vi "SubVI_SingleWrite.vi"() -> ()   [LabVIEW 2022 SP3, in "ADS_Library.lvlib"]
uses:
  ADS_Library.lvlib
  <userlib>/Beckhoff-LabVIEW-Interface/_DependsOn/Base/Write/Write Sync.vi
panel:
  in  "Ads Write Data":variant
  out "Write Status":bool
  out "SymbolName":string
  out "error out":errorcluster
  in  "error in":errorcluster
  in  "String":string
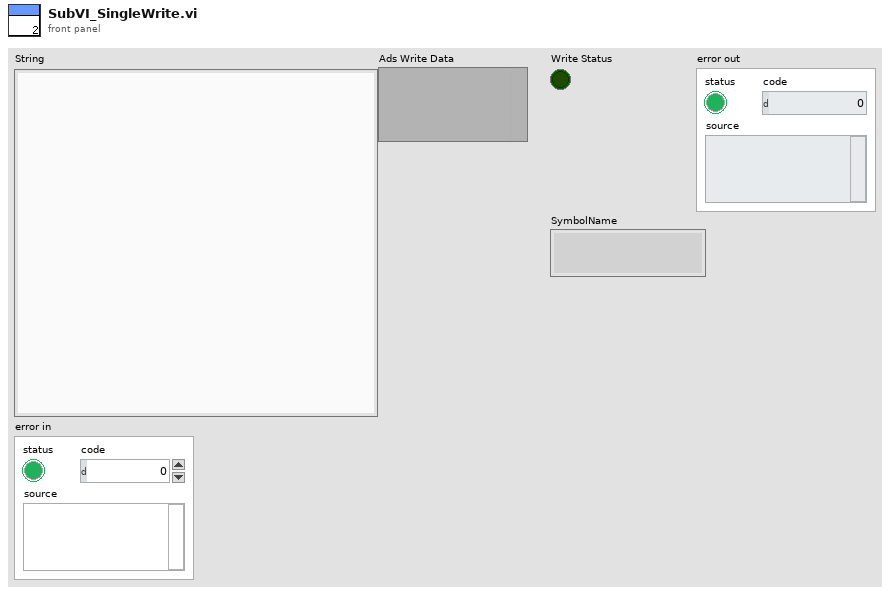
[diagram p1: front panel]
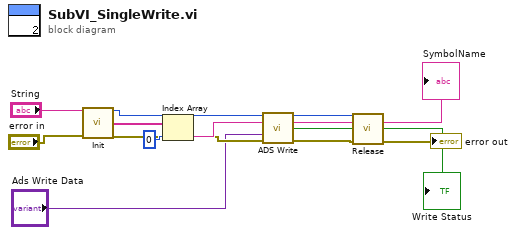
[diagram p0: block diagram]
diagram:
  n1 = call <userlib>:"Init.vi"("XMLDescription"="String", "error in (no error)"="error in") -> ("Handle"=w8:u32, "ReadGrpSymbols"=w12:string[], "error out"=w6:errorcluster)  [unwired: 9 in, 2 out]
  n2 = Index Array(array=w12, index=0) -> (element=w7:string)
  n3 = call-poly <userlib>:"ADS Write.vi"("Handle"=w8, "SymbolName"=w7, "Ads Write Data"="Ads Write Data", "error in (no error)"=w6) -> ("Handle"=w4:u32, "SymbolName"=→"SymbolName":string, "Write Status"=→"Write Status":bool, "error out"=w5:errorcluster)  [unwired: 8 in]
  n4 = call <userlib>:"Release.vi"("Handle"=w4, "error in (no error)"=w5) -> ("error out"=→"error out":errorcluster)  [unwired: 13 in]
